vi "List Sections.vi"(8 "error in (no error)":errorcluster, 11 "Ini Path in":path) -> (0 "error out":errorcluster, 2 "Sections":string[](array[string]), 3 "Ini Path out":path)   [LabVIEW 2018, in "Config.lvlib"]
uses:
  Config.lvlib
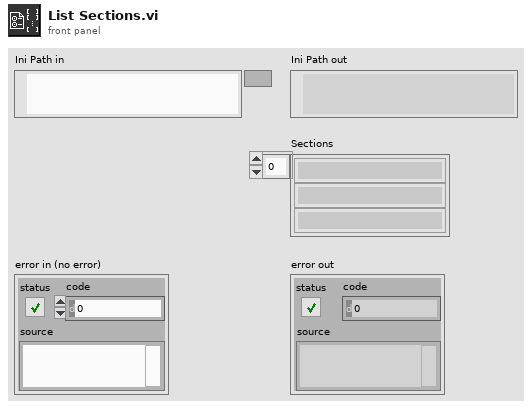
[diagram p1: front panel]
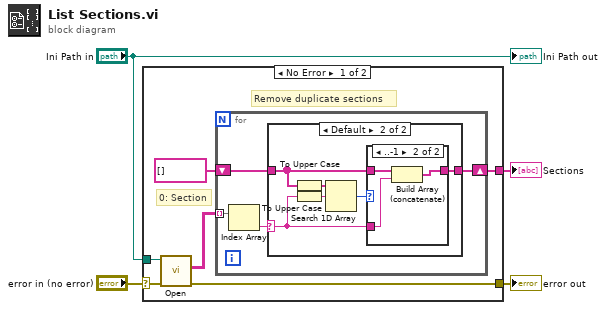
[diagram p0: block diagram]
diagram:
  n1 = case shown="No Error" "error in (no error)" {
    selector: "error in (no error)" -> [w10 w26]
    tunnel: [w9 w26] -> w2
    tunnel: "Ini Path in" -> [w8 _]
    tunnel: [w5 _] -> w1
    frame No Error {
      # "0: Section"
      # "Remove duplicate sections"
      n2 = call "Open.vi"("error in (no error)"=w10, "Ini Path in"=w8) -> ("error out"=w9:errorcluster, "skvc out"=w6:string[][])  [unwired: 6 in, 2 out]
      n3 = for {
        tunnel: w6 -> [w14] mode=indexing
        shift-right: [w13] -> w5
        shift-left: string[] [] -> [w12]
        n4 = Index Array(array=w14) -> (element=w11:string)  [unwired: 1 in]
        n5 = case shown="Default" w11 {
          selector: w11 -> [_ w16]
          tunnel: [w15 w18] -> w13
          tunnel: w12 -> [w15 w17]
          frame "" {
          }
          frame Default {
            n6 = To Upper Case(1:w17) -> (0:w21:string[])
            n7 = To Upper Case(1:w16) -> (0:w20:string)
            n8 = Search 1D Array(1D array=w21, element=w20) -> (index of element=w19:i32)  [unwired: 1 in]
            n9 = case shown="..-1" w19 {
              tunnel: [w22 w24] -> w18
              tunnel: w17 -> [w22 w25]
              tunnel: w16 -> [_ w23]
              frame 0.. {
              }
              frame ..-1 {
                n10 = Build Array (concatenate)(w25, w23) -> (w24:string[])
              }
            }
          }
        }
      }
    }
    frame Error {
    }
  }
  "error out" <- w2
  "Sections" <- w1
  "Ini Path out" <- "Ini Path in"
